vi "Get Magnet Field.vi"(4 "Axis":T1, 8 "error in (no error)":errorcluster, 11 "instrument.PPMS2 in":refnum<class "instrument.PPMS2.lvclass">) -> (0 "error out":errorcluster, 1 "Status":variant, 2 "B Field (T)":dbl, 3 "instrument.PPMS2 out":refnum<class "instrument.PPMS2.lvclass">)   [LabVIEW 2016, in "instrument.PPMS2.lvclass"]
uses:
  instrument.PPMS2.lvclass
  <userlib>/LevyLab/Levylab Instruments/Instrument Types/Cryostat/Typedefs/Magnet Axis--Enum.ctl
  Typedefs/Magnet Status--PPMS2--cluster.ctl
  Typedefs/Magnet Status--PPMS2--ring.ctl
  <userlib>/LevyLab/Levylab Instruments/Instrument Types/Cryostat/Instrument.Cryostat.lvclass
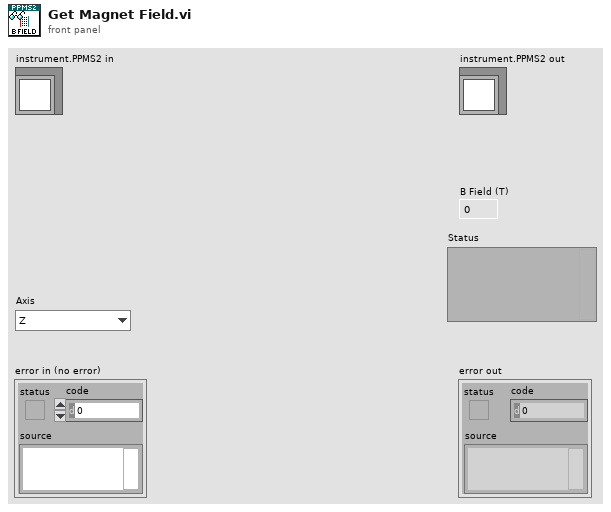
[diagram p1: front panel]
types:
  T1 = typedef "Instrument.Cryostat.lvclass/Magnet Axis--Enum.ctl" = enum16{"Z", "X", "Y"}
  T2 = typedef "instrument.PPMS2.lvclass/Magnet Status--PPMS2--cluster.ctl" = cluster{"Field (Oe)":dbl, "Field Status":T3}
  T3 = typedef "instrument.PPMS2.lvclass/Magnet Status--PPMS2--ring.ctl" = i32
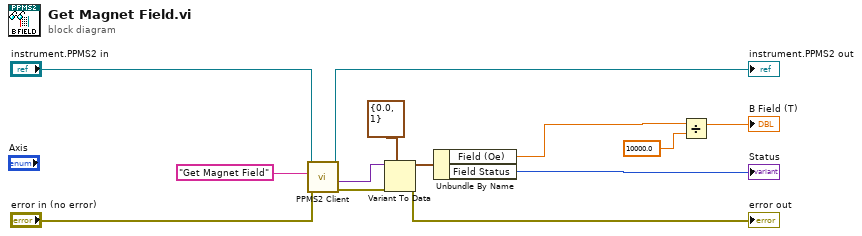
[diagram p0: block diagram]
diagram:
  n1 = call "PPMS2 Client.vi"("error in (no error)"="error in (no error)", "Command"="Get Magnet Field", "instrument.PPMS2 in"="instrument.PPMS2 in") -> ("error out"=w2:errorcluster, "Data out"=w3:variant, "instrument.PPMS2 out"=→"instrument.PPMS2 out":refnum<class "instrument.PPMS2.lvclass">)  [unwired: 5 in, 1 out]
  n2 = Variant To Data(error in=w2, type=T2 {"Field (Oe)"=0.0, "Field Status"=1} ("cluster"), Variant=w3) -> (data=w4:T2, error out=→"error out":errorcluster)
  n3 = Unbundle By Name(w4) -> ("Field (Oe)"=w7:dbl, "Field Status"=→"Status":T3)
  n4 = Divide(x=w7, y=10000.0) -> (x/y=→"B Field (T)":dbl)
